vi "test Receive Stop Flag.vi"(8 "error in (no error)":errorcluster, 11 "TestCase in":refnum<class "Test Network Stream Transmission.lvclass">) -> (0 "error out":errorcluster, 3 "TestCase out":refnum<class "Test Network Stream Transmission.lvclass">)   [LabVIEW 2020, in "Test Network Stream Transmission.lvclass"]
uses:
  Test Network Stream Transmission.lvclass
  <vilib>/addons/_JKI Toolkits/VI Tester/TestCase.llb/TestCase.lvclass
  <vilib>/ActorFramework/LastAck/Last Ack.lvclass
  Source/Protocols/Network Stream Strategy/Network Stream Initiator/Network Stream Initiator.lvclass
  Source/Abstract Classes/Cipher/Cipher.lvclass
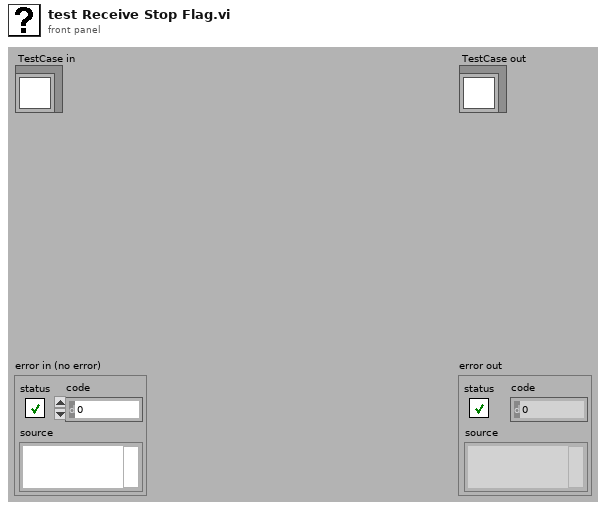
[diagram p1: front panel]
types:
  T1 = cluster{"Last Ack":refnum<class "Last Ack.lvclass">, "priority":i32}
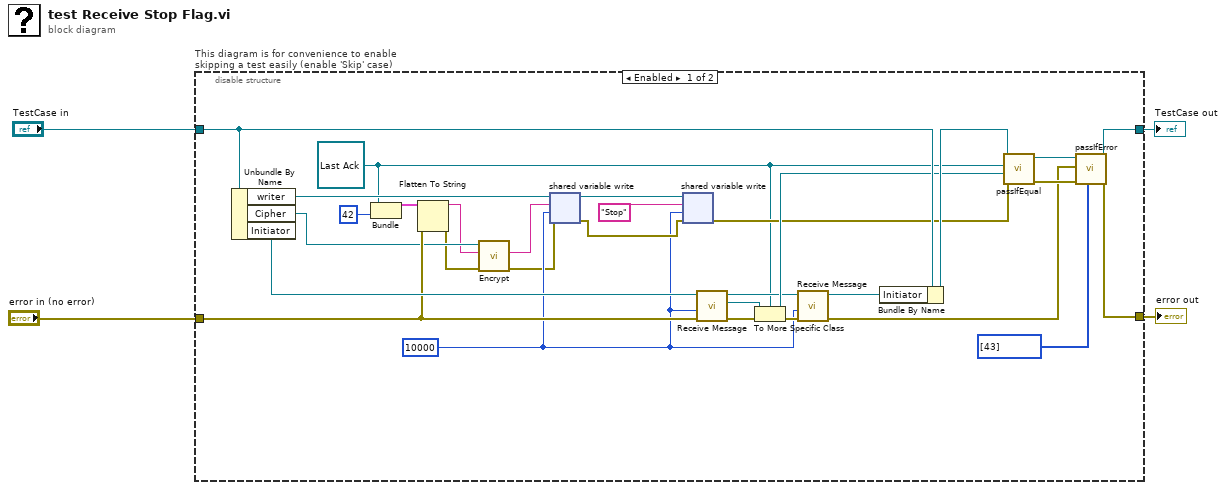
[diagram p0: block diagram]
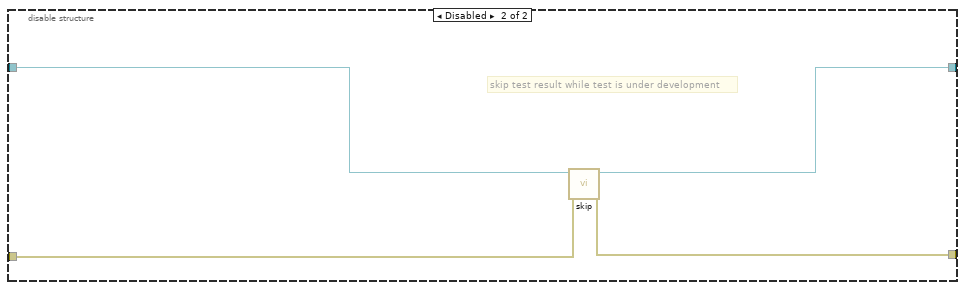
[diagram p2: hidden frame]
diagram:
  n1 = disable-structure "This diagram is for convenience to enable skipping a test easily (enable 'Skip' case)" shown="Enabled" {
    disable-tunnel: "TestCase in" -> [w32 w38]
    disable-tunnel: [w23 w36] -> w1
    disable-tunnel: [w19 w37] -> w3
    disable-tunnel: "error in (no error)" -> [w13 w35]
    frame Enabled {
      w10 = 10000 ("timeout ms (-1)")
      w18 = refnum<class "Last Ack.lvclass"> refnum ("Last Ack")
      n2 = Unbundle By Name(w32) -> ("writer"=w34:refnum<k21>, "Cipher"=w9:refnum<class "Cipher.lvclass">, "Initiator"=w15:refnum<class "Network Stream Initiator.lvclass">)
      n3 = Bundle("Last Ack"=w18, "priority"=42) -> (w17:T1)  [unwired: 1 in]
      n4 = Flatten To String(anything=w17, error in (no error)=w13) -> (data string=w5:string, error out=w8:errorcluster)  [unwired: 2 in, 1 out]
      n5 = call-dynamic "Encrypt.vi"("error in (no error)"=w8, "Plaintext"=w5, "Cipher in"=w9) -> ("error out"=w7:errorcluster, "Cyphertext"=w6:string)  [unwired: 6 in, 1 out]
      n6 = shared-variable-write(w34, w7, w6, w10) -> (w29:refnum<k21>, w11:errorcluster)  [unwired: 1 out]
      n7 = shared-variable-write(w29, w11, "Stop" ("data in"), w10) -> (w25:errorcluster)  [unwired: 2 out]
      n8 = call-dynamic "Receive Message.vi"("error in (no error)"=w13, "timeout ms (-1)"=w10, "Network Stream in"=w15) -> ("error out"=w33:errorcluster, "Message"=w12:refnum<class "Message.lvclass">, "Network Stream out"=w28:refnum<class "Network Stream Initiator.lvclass">)  [unwired: 4 in, 2 out]
      n9 = To More Specific Class(target class=w18, reference=w12, error in=w33) -> (specific class reference=w30:refnum<class "Last Ack.lvclass">, error out=w27:errorcluster)
      n10 = call-dynamic "Receive Message.vi"("error in (no error)"=w27, "timeout ms (-1)"=w10, "Network Stream in"=w28) -> ("error out"=w20:errorcluster, "Network Stream out"=w26:refnum<class "Network Stream Initiator.lvclass">)  [unwired: 4 in, 3 out]
      n11 = Bundle By Name(cluster=w32, "Initiator"=w26) -> (w31:refnum<class "Test Network Stream Transmission.lvclass">)
      n12 = call-dynamic "passIfEqual.vi"("error in (no error)"=w25, "y"=w30, "x"=w18, "TestCase in"=w31) -> ("error out"=w21:errorcluster, "TestCase out"=w24:refnum<class "Test Network Stream Transmission.lvclass">)  [unwired: 6 in]
      n13 = call-dynamic "passIfError.vi"("passing error codes (default = any error code)"=i32[] [43], "error in (no error)"=w21, "error"=w20, "TestCase in"=w24) -> ("error out"=w19:errorcluster, "TestCase out"=w23:refnum<class "Test Network Stream Transmission.lvclass">)  [unwired: 6 in]
    }
    frame Disabled {
      # "skip test result while test is under development"
      n14 = call <vilib>:"skip.vi"("error in (no error)"=w35, "TestCase in"=w38) -> ("error out"=w37:errorcluster, "TestCase out"=w36:refnum<class "Test Network Stream Transmission.lvclass">)  [unwired: 8 in]
    }
  }
  "error out" <- w3
  "TestCase out" <- w1
